vi "Alpha Ver 1.0.vi"() -> ()   [LabVIEW 2015]
uses:
  <instrlib>/Keithley 622x LV 2009/Utility/Typedefs/KE622x -- Instrument Type.ctl
  <instrlib>/Keithley 622x LV 2009/Keithley 622x.lvlib
panel:
  in  "Ring":u16(ring)
  in  "Low Measure":u16(ring)
  in  "Interval":dbl
  in  "Ranging":string(combo)="BEST"
  in  "Count":dbl
  in  "Source Delay":dbl
  in  "Width":dbl
  in  "Low Level":dbl min=-0.105 max=0.105
  in  "High Level":dbl min=-0.105 max=0.105
  out "2182A \nconnected ?":string
  in  "STOP":bool
  out "Measurement\nUnits":string
  out "2182A Voltage \nRange":string
  out "error out":errorcluster
  # "Pulse Measurement System"
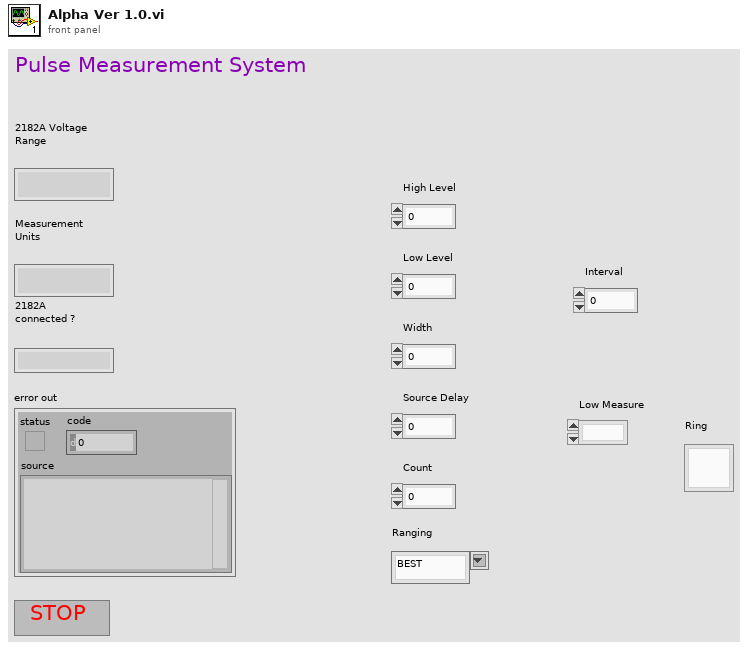
[diagram p1: front panel]
types:
  T1 = typedef "Keithley 622x.lvlib/KE622x -- Instrument Type.ctl" = enum16{"KE6220", "KE6221"}
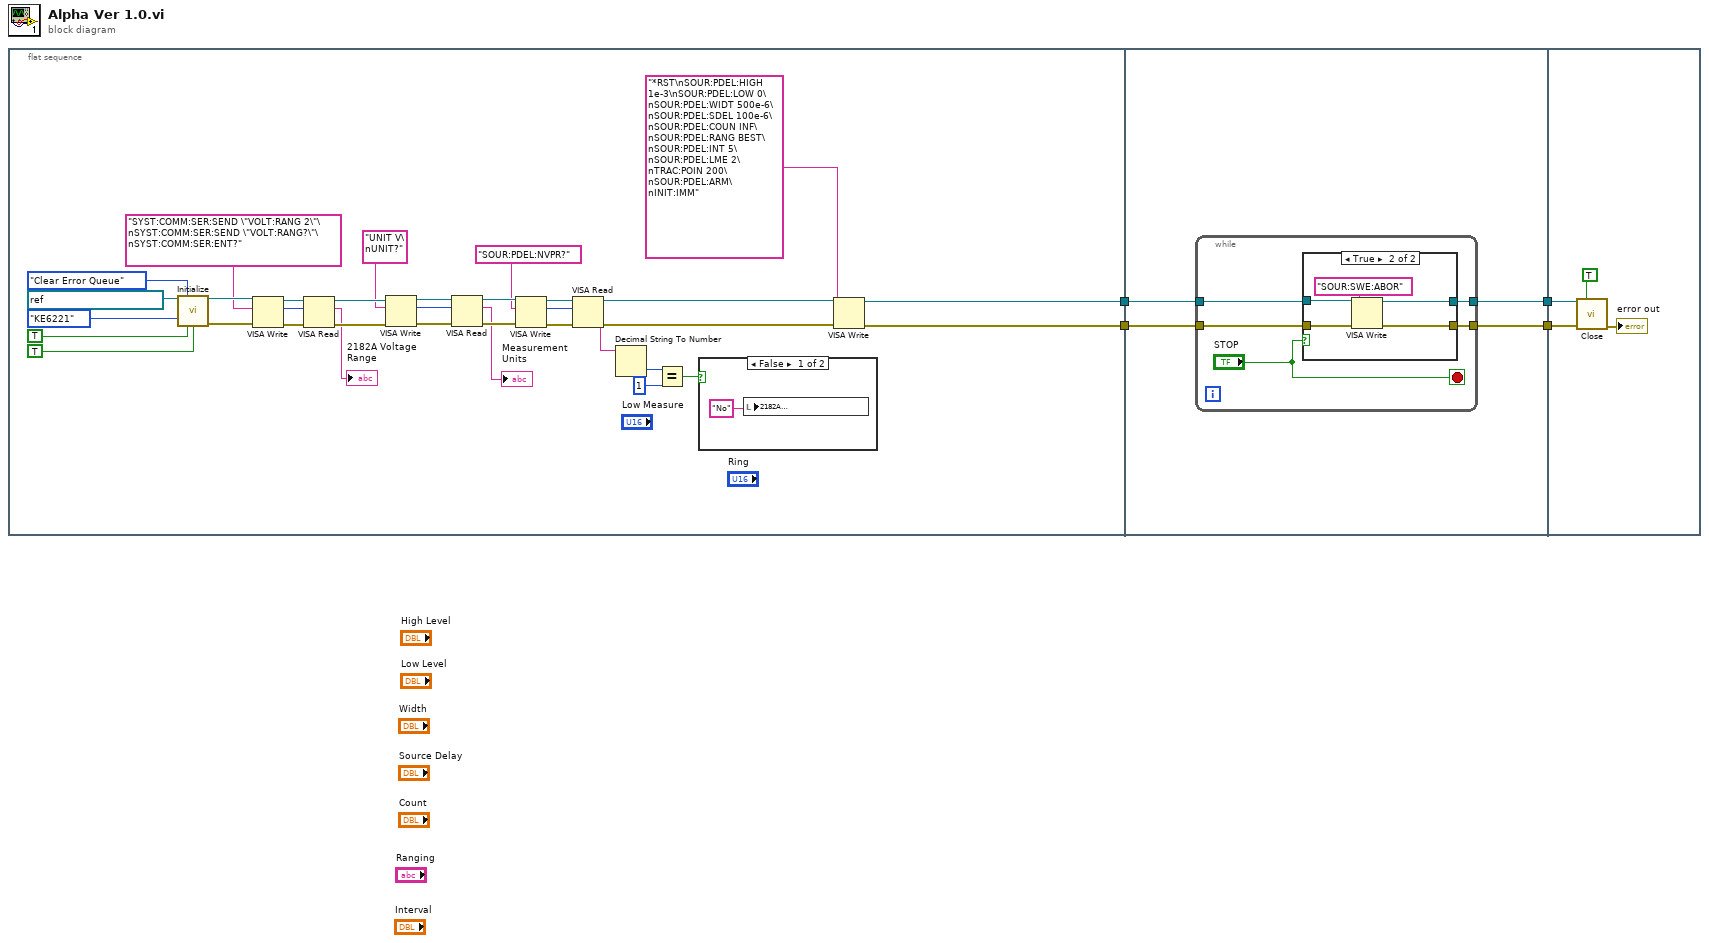
[diagram p0: block diagram]
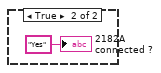
[diagram p2: hidden frame]
diagram:
  n1 = flat-sequence {
    tunnel: [w10] -> w4
    tunnel: [w9] -> w3
    tunnel: w4 -> [w44]
    tunnel: w3 -> [w43]
    tunnel: [w42] -> w2
    tunnel: [w41] -> w1
    tunnel: w2 -> [w58]
    tunnel: w1 -> [w57]
    frame #0 {
      n2 = call <instrlib>:"Initialize.vi"("VISA resource name"=refnum<visa-resource-name> "Keithley_6221_2182A", "Error Queue Option"=enum16{"Clear Error Queue", "Error Query"}."Clear Error Queue", "Instrument Type"=KE622x_--_Instrument_Type."KE6221", "ID Query? (T)"=TRUE, "Reset? (T)"=TRUE) -> ("VISA resource name out"=w35:refnum<visa-resource-name>, "error out"=w34:errorcluster)  [unwired: 9 in]
      n3 = VISA Write(VISA resource name=w35, write buffer="SYST:COMM:SER:SEND \"VOLT:RANG 2\"\nSYST:COMM:SER:SEND \"VOLT:RANG?\"\nSYST:COMM:SER:ENT?", error in (no error)=w34) -> (VISA resource name out=w29:refnum<visa-resource-name>, return count=w30:u32, error out=w28:errorcluster)
      n4 = VISA Read(VISA resource name=w29, byte count=w30, error in (no error)=w28) -> (VISA resource name out=w25:refnum<visa-resource-name>, read buffer=→"2182A Voltage \nRange":string, error out=w27:errorcluster)  [unwired: 1 out]
      n5 = VISA Write(VISA resource name=w25, write buffer="UNIT V\nUNIT?", error in (no error)=w27) -> (VISA resource name out=w21:refnum<visa-resource-name>, return count=w22:u32, error out=w23:errorcluster)
      n6 = VISA Read(VISA resource name=w21, byte count=w22, error in (no error)=w23) -> (VISA resource name out=w18:refnum<visa-resource-name>, read buffer=→"Measurement\nUnits":string, error out=w20:errorcluster)  [unwired: 1 out]
      n7 = VISA Write(VISA resource name=w18, write buffer="SOUR:PDEL:NVPR?", error in (no error)=w20) -> (VISA resource name out=w14:refnum<visa-resource-name>, return count=w15:u32, error out=w16:errorcluster)
      n8 = VISA Read(VISA resource name=w14, byte count=w15, error in (no error)=w16) -> (VISA resource name out=w12:refnum<visa-resource-name>, read buffer=w7:string, error out=w13:errorcluster)  [unwired: 1 out]
      n9 = Decimal String To Number(string=w7) -> (number=w6:i32)  [unwired: 2 in, 1 out]
      n10 = Equal?(x=w6, y=1) -> (x = y?=w8:bool)
      n11 = case shown="False" w8 {
        frame False {
          n12 = local write "2182A \nconnected ?"("No" ("2182A \nconnected ?")) -> ()
        }
        frame True {
          "2182A \nconnected ?" <- "Yes" ("2182A \nconnected ?")
        }
      }
      n13 = VISA Write(VISA resource name=w12, write buffer="*RST\nSOUR:PDEL:HIGH 1e-3\nSOUR:PDEL:LOW 0\nSOUR:PDEL:WIDT 500e-6\nSOUR:PDEL:SDEL 100e-6\nSOUR:PDEL:COUN INF\nSOUR:PDEL:RANG BEST\nSOUR:PDEL:INT 5\nSOUR:PDEL:LME 2\nTRAC:POIN 200\nSOUR:PDEL:ARM\nINIT:IMM", error in (no error)=w13) -> (VISA resource name out=w10:refnum<visa-resource-name>, error out=w9:errorcluster)  [unwired: 1 out]
    }
    frame #1 {
      n14 = while {
        tunnel: w44 -> [w49]
        tunnel: w43 -> [w48]
        tunnel: [w46] -> w42
        tunnel: [w45] -> w41
        stop <- "STOP" stop-if-true
        n15 = case shown="True" "STOP" {
          tunnel: w49 -> [w50 w55]
          tunnel: w48 -> [w51 w54]
          tunnel: [w50 w53] -> w46
          tunnel: [w51 w52] -> w45
          frame False {
          }
          frame True {
            n16 = VISA Write(VISA resource name=w55, write buffer="SOUR:SWE:ABOR", error in (no error)=w54) -> (VISA resource name out=w53:refnum<visa-resource-name>, error out=w52:errorcluster)  [unwired: 1 out]
          }
        }
      }
    }
    frame #2 {
      n17 = call <instrlib>:"Close.vi"("VISA resource name"=w58, "Query For SCPI Errors? (T)"=TRUE, "error in (no error)"=w57) -> ("error out"=→"error out":errorcluster)  [unwired: 12 in]
    }
  }
